vi "Finish.vi"   [LabVIEW 2018]
doc: "This VI is called just before exiting. It is expected to close I/O refnum, save collected data, etc."
uses:
  RefNums_DriverStation.vi
  RefNums_Actuators.vi
  RefNums_Sensors.vi
  <vilib>/Rock Robotics/WPI/Utilities/WPI_GetSetVariantRefNum.vi
types:
  T1 = typedef "WPI_AnalogChannelDevRef.ctl" = cluster{"DevStatus":errorcluster, "Analog Channel":T2}
  T2 = typedef "FPGA_AIChannel.ctl" = enum8{"AI 0", "AI 1", "AI 2", "AI 3", "AI MXP 0", "AI MXP 1", "AI MXP 2", "AI MXP 3", "Invalid"}
  T3 = typedef "WPI_RobotDriveDevRef.ctl" = cluster{"DevStatus":errorcluster, "Motors[]":T4[], "Square Inputs":bool, "Max Output":dbl}
  T4 = typedef "WPI_MotorControlDeviceRef.ctl" = cluster{"DeviceStatus":errorcluster, "Type":T5, "PWM":cluster{"PWM Channel":T6, "DeadBand":T7}, "CAN":cluster{"Device Number":u8, "SetOutput VI Ref":variant, "GetOutput VI Ref":variant, "Enable VI Ref":variant, "Disable VI Ref":variant, "Data":variant}, "Invert":bool, "DIO PWM":cluster{"PWM \"Enable\" Channel":T6, "DIOChannel":T8, "PWM Rate":dbl}}
  T5 = typedef "WPI_MotorControlType.ctl" = enum16{"PWM", "CAN", "DIO PWM"}
  T6 = typedef "FPGA_DIOPWMChannel.ctl" = enum8{"PWM 0", "PWM 1", "PWM 2", "PWM 3", "PWM 4", "PWM 5", "PWM 6", "PWM 7", "PWM 8", "PWM 9", "PWM MXP 0", "PWM MXP 1", "PWM MXP 2", "PWM MXP 3", "PWM MXP 4", "PWM MXP 5", "PWM MXP 6", "PWM MXP 7", "PWM MXP 8", "PWM MXP 9", "Invalid"}
  T7 = typedef "WPI_PWMDeadband.ctl" = cluster{"Name":string, "maxPositivePwm":i32, "minPositivePwm":i32, "centerPwm":i32, "maxNegativePwm":i32, "minNegativePwm":i32, "angularRange":u16}
  T8 = typedef "FPGA_DIOChannel.ctl" = enum8{"DIO 0", "DIO 1", "DIO 2", "DIO 3", "DIO 4", "DIO 5", "DIO 6", "DIO 7", "DIO 8", "DIO 9", "DIO MXP 0", "DIO MXP 1", "DIO MXP 2", "DIO MXP 3", "DIO MXP 4", "DIO MXP 5", "DIO MXP 6", "DIO MXP 7", "DIO MXP 8", "DIO MXP 9", "DIO MXP 10", "DIO MXP 11", "DIO MXP 12", "DIO MXP 13", "DIO MXP 14", "DIO MXP 15", "SPI Port CS1", "SPI Port CS2", "SPI Port CS3", "SPI Port MISO", "SPI Port MOSI", "Invalid"}
  T9 = typedef "WPI_ServoDeviceRef.ctl" = cluster{"DeviceStatus":errorcluster, "PWM Channel":T6, "DeadBand":T7}
  T10 = typedef "WPI_SolenoidDevRef.ctl" = cluster{"DevStatus":errorcluster, "Pneumatics Control Module":u8, "Forward Solenoid Channel":T11, "Reverse Solenoid Channel":T11}
  T11 = typedef "WPI_SolenoidChannel.ctl" = enum8{"Solenoid 0", "Solenoid 1", "Solenoid 2", "Solenoid 3", "Solenoid 4", "Solenoid 5", "Solenoid 6", "Solenoid 7", "Invalid"}
  T12 = typedef "WPI_JoystickDevRef.ctl" = cluster{"Device":T13}
  T13 = typedef "WPI_JoystickDeviceEnum.ctl" = enum16{"USB 0", "USB 1", "USB 2", "USB 3", "USB 4", "USB 5"}
  T14 = typedef "WPI_CompressorDevRef.ctl" = cluster{"DevStatus":errorcluster, "Pneumatics Control Module":u8}
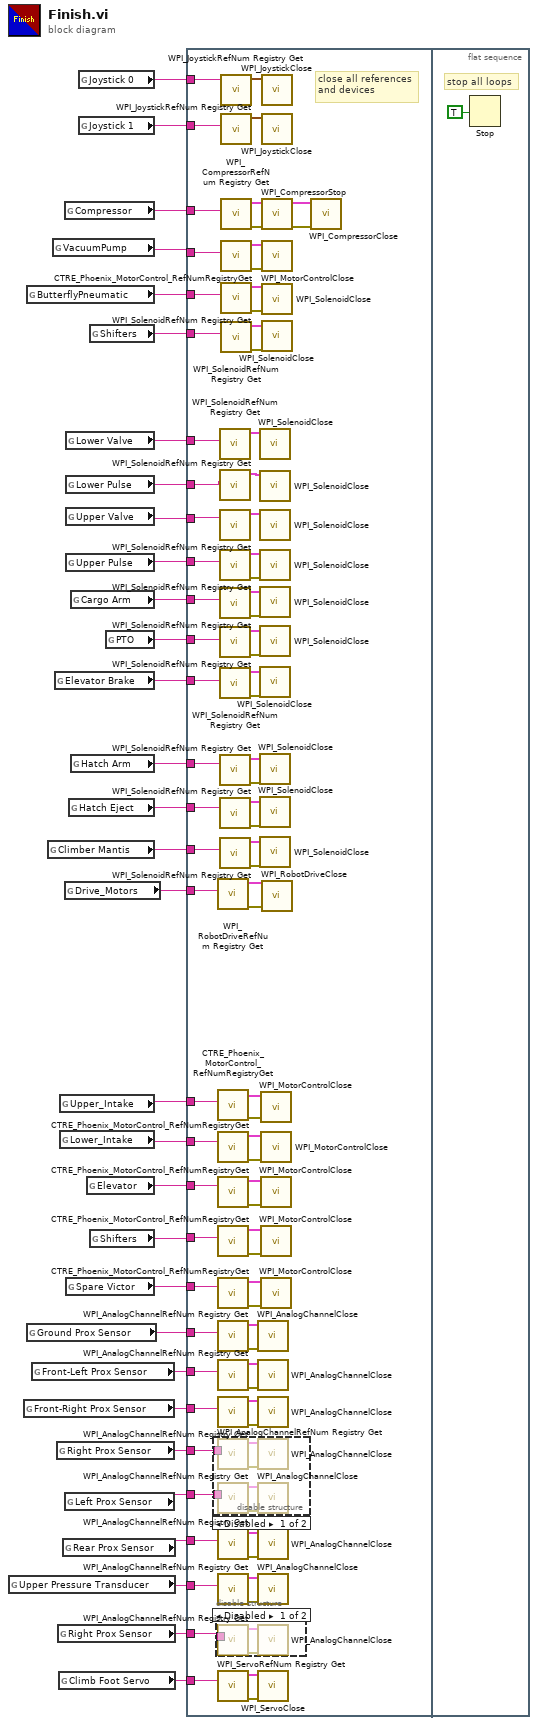
[diagram p0: block diagram]
diagram:
  n1 = global read "RefNums_Sensors.vi" "Upper Pressure Transducer"() -> (w18:string)
  n2 = global read "RefNums_Sensors.vi" "Front-Right Prox Sensor"() -> (w5:string)
  n3 = global read "RefNums_Actuators.vi" "ButterflyPneumatic"() -> (w28:string)
  n4 = global read "RefNums_Sensors.vi" "Ground Prox Sensor"() -> (w4:string)
  n5 = global read "RefNums_Sensors.vi" "Front-Left Prox Sensor"() -> (w6:string)
  n6 = global read "RefNums_Actuators.vi" "Climber Mantis"() -> (w10:string)
  n7 = global read "RefNums_Actuators.vi" "VacuumPump"() -> (w26:string)
  n8 = global read "RefNums_Actuators.vi" "Elevator Brake"() -> (w13:string)
  n9 = global read "RefNums_Sensors.vi" "Right Prox Sensor"() -> (w20:string)
  n10 = global read "RefNums_Sensors.vi" "Right Prox Sensor"() -> (w3:string)
  n11 = global read "RefNums_Actuators.vi" "Climb Foot Servo"() -> (w1:string)
  n12 = global read "RefNums_Actuators.vi" "Upper_Intake"() -> (w23:string)
  n13 = global read "RefNums_Actuators.vi" "Lower_Intake"() -> (w22:string)
  n14 = global read "RefNums_Sensors.vi" "Rear Prox Sensor"() -> (w17:string)
  n15 = global read "RefNums_Actuators.vi" "Compressor"() -> (w29:string)
  n16 = global read "RefNums_Actuators.vi" "Drive_Motors"() -> (w2:string)
  n17 = global read "RefNums_Sensors.vi" "Left Prox Sensor"() -> (w19:string)
  n18 = global read "RefNums_Actuators.vi" "Lower Valve"() -> (w8:string)
  n19 = global read "RefNums_Actuators.vi" "Lower Pulse"() -> (w7:string)
  n20 = global read "RefNums_Actuators.vi" "Upper Valve"() -> (w9:string)
  n21 = global read "RefNums_Actuators.vi" "Upper Pulse"() -> (w25:string)
  n22 = global read "RefNums_Actuators.vi" "Spare Victor"() -> (w15:string)
  n23 = global read "RefNums_Actuators.vi" "Hatch Eject"() -> (w11:string)
  n24 = global read "RefNums_Actuators.vi" "Cargo Arm"() -> (w24:string)
  n25 = global read "RefNums_Actuators.vi" "Hatch Arm"() -> (w12:string)
  n26 = global read "RefNums_DriverStation.vi" "Joystick 0"() -> (w30:string)
  n27 = global read "RefNums_DriverStation.vi" "Joystick 1"() -> (w31:string)
  n28 = global read "RefNums_Actuators.vi" "Elevator"() -> (w21:string)
  n29 = global read "RefNums_Actuators.vi" "Shifters"() -> (w27:string)
  n30 = global read "RefNums_Actuators.vi" "Shifters"() -> (w16:string)
  n31 = global read "RefNums_Actuators.vi" "PTO"() -> (w14:string)
  n32 = flat-sequence {
    tunnel: w31 -> [w114]
    tunnel: w30 -> [w115]
    tunnel: w29 -> [w111]
    tunnel: w28 -> [w110]
    tunnel: w27 -> [w105]
    tunnel: w26 -> [w104]
    tunnel: w25 -> [w102]
    tunnel: w24 -> [w99]
    tunnel: w23 -> [w97]
    tunnel: w22 -> [w95]
    tunnel: w21 -> [w93]
    tunnel: w20 -> [w92]
    tunnel: w19 -> [w77]
    tunnel: w17 -> [w76]
    tunnel: w18 -> [w75]
    tunnel: w16 -> [w72]
    tunnel: w15 -> [w70]
    tunnel: w14 -> [w64]
    tunnel: w13 -> [w63]
    tunnel: w12 -> [w56]
    tunnel: w11 -> [w55]
    tunnel: w10 -> [w54]
    tunnel: w9 -> [w50]
    tunnel: w8 -> [w49]
    tunnel: w7 -> [w48]
    tunnel: w6 -> [w43]
    tunnel: w5 -> [w42]
    tunnel: w4 -> [w39]
    tunnel: w3 -> [w38]
    tunnel: w2 -> [w35]
    tunnel: w1 -> [w34]
    frame #0 {
      # "close all references\nand devices"
      n33 = disable-structure shown="Disabled" {
        disable-tunnel: w92 -> [w123 _]
        disable-tunnel: w77 -> [w119 _]
        frame Disabled {
          n34 = call <vilib>:"WPI_AnalogChannelRefNum Registry Get.vi"("refnum name"=w123) -> ("error out"=w122:errorcluster, "AIDeviceRef"=w124:T1)  [unwired: 9 in]
          n35 = call <vilib>:"WPI_AnalogChannelRefNum Registry Get.vi"("refnum name"=w119) -> ("error out"=w120:errorcluster, "AIDeviceRef"=w121:T1)  [unwired: 9 in]
          n36 = call <vilib>:"WPI_AnalogChannelClose.vi"("error in (no error)"=w122, "AIDeviceRef"=w124) -> ()  [unwired: 9 in, 1 out]
          n37 = call <vilib>:"WPI_AnalogChannelClose.vi"("error in (no error)"=w120, "AIDeviceRef"=w121) -> ()  [unwired: 9 in, 1 out]
        }
        frame Enabled {
        }
      }
      n38 = disable-structure shown="Disabled" {
        disable-tunnel: w38 -> [w116 _]
        frame Disabled {
          n39 = call <vilib>:"WPI_AnalogChannelRefNum Registry Get.vi"("refnum name"=w116) -> ("error out"=w118:errorcluster, "AIDeviceRef"=w117:T1)  [unwired: 9 in]
          n40 = call <vilib>:"WPI_AnalogChannelClose.vi"("error in (no error)"=w118, "AIDeviceRef"=w117) -> ()  [unwired: 9 in, 1 out]
        }
        frame Enabled {
        }
      }
      n41 = call <vilib>:"WPI_RobotDriveRefNum Registry Get.vi"("refnum name"=w35) -> ("error out"=w37:errorcluster, "RobotDriveDevRef"=w36:T3)  [unwired: 9 in]
      n42 = call <vilib>:"CTRE_Phoenix_MotorControl_RefNumRegistryGet.vi"("refnum name"=w97) -> ("error out"=w89:errorcluster, "PhoenixMotorControlDevRef"=w98:T4)  [unwired: 9 in]
      n43 = call <vilib>:"CTRE_Phoenix_MotorControl_RefNumRegistryGet.vi"("refnum name"=w95) -> ("error out"=w90:errorcluster, "PhoenixMotorControlDevRef"=w96:T4)  [unwired: 9 in]
      n44 = call <vilib>:"CTRE_Phoenix_MotorControl_RefNumRegistryGet.vi"("refnum name"=w93) -> ("error out"=w91:errorcluster, "PhoenixMotorControlDevRef"=w94:T4)  [unwired: 9 in]
      n45 = call <vilib>:"CTRE_Phoenix_MotorControl_RefNumRegistryGet.vi"("refnum name"=w72) -> ("error out"=w74:errorcluster, "PhoenixMotorControlDevRef"=w73:T4)  [unwired: 9 in]
      n46 = call <vilib>:"CTRE_Phoenix_MotorControl_RefNumRegistryGet.vi"("refnum name"=w70) -> ("error out"=w71:errorcluster, "PhoenixMotorControlDevRef"=w69:T4)  [unwired: 9 in]
      n47 = call <vilib>:"WPI_AnalogChannelRefNum Registry Get.vi"("refnum name"=w39) -> ("error out"=w40:errorcluster, "AIDeviceRef"=w41:T1)  [unwired: 9 in]
      n48 = call <vilib>:"WPI_AnalogChannelRefNum Registry Get.vi"("refnum name"=w43) -> ("error out"=w44:errorcluster, "AIDeviceRef"=w45:T1)  [unwired: 9 in]
      n49 = call <vilib>:"WPI_AnalogChannelRefNum Registry Get.vi"("refnum name"=w42) -> ("error out"=w46:errorcluster, "AIDeviceRef"=w47:T1)  [unwired: 9 in]
      n50 = call <vilib>:"WPI_AnalogChannelRefNum Registry Get.vi"("refnum name"=w76) -> ("error out"=w80:errorcluster, "AIDeviceRef"=w81:T1)  [unwired: 9 in]
      n51 = call <vilib>:"WPI_AnalogChannelRefNum Registry Get.vi"("refnum name"=w75) -> ("error out"=w78:errorcluster, "AIDeviceRef"=w79:T1)  [unwired: 9 in]
      n52 = call <vilib>:"WPI_ServoRefNum Registry Get.vi"("refnum name"=w34) -> ("error out"=w33:errorcluster, "ServoDeviceRef"=w32:T9)  [unwired: 9 in]
      n53 = call <vilib>:"WPI_SolenoidRefNum Registry Get.vi"("refnum name"=w49) -> ("SolenoidDevRef"=w53:T10)  [unwired: 9 in, 1 out]
      n54 = call <vilib>:"WPI_SolenoidRefNum Registry Get.vi"("refnum name"=w48) -> ("SolenoidDevRef"=w52:T10)  [unwired: 9 in, 1 out]
      n55 = call <vilib>:"WPI_SolenoidRefNum Registry Get.vi"("refnum name"=w50) -> ("SolenoidDevRef"=w51:T10)  [unwired: 9 in, 1 out]
      n56 = call <vilib>:"WPI_SolenoidRefNum Registry Get.vi"("refnum name"=w102) -> ("error out"=w87:errorcluster, "SolenoidDevRef"=w101:T10)  [unwired: 9 in]
      n57 = call <vilib>:"WPI_SolenoidRefNum Registry Get.vi"("refnum name"=w99) -> ("error out"=w88:errorcluster, "SolenoidDevRef"=w100:T10)  [unwired: 9 in]
      n58 = call <vilib>:"WPI_SolenoidRefNum Registry Get.vi"("refnum name"=w64) -> ("error out"=w67:errorcluster, "SolenoidDevRef"=w68:T10)  [unwired: 9 in]
      n59 = call <vilib>:"WPI_SolenoidRefNum Registry Get.vi"("refnum name"=w63) -> ("error out"=w65:errorcluster, "SolenoidDevRef"=w66:T10)  [unwired: 9 in]
      n60 = call <vilib>:"WPI_SolenoidRefNum Registry Get.vi"("refnum name"=w56) -> ("error out"=w61:errorcluster, "SolenoidDevRef"=w62:T10)  [unwired: 9 in]
      n61 = call <vilib>:"WPI_SolenoidRefNum Registry Get.vi"("refnum name"=w55) -> ("error out"=w59:errorcluster, "SolenoidDevRef"=w60:T10)  [unwired: 9 in]
      n62 = call <vilib>:"WPI_SolenoidRefNum Registry Get.vi"("refnum name"=w54) -> ("error out"=w57:errorcluster, "SolenoidDevRef"=w58:T10)  [unwired: 9 in]
      n63 = call <vilib>:"WPI_JoystickRefNum Registry Get.vi"("refnum name"=w115) -> ("JoystickDevRef"=w112:T12)  [unwired: 9 in, 1 out]
      n64 = call <vilib>:"WPI_JoystickRefNum Registry Get.vi"("refnum name"=w114) -> ("JoystickDevRef"=w113:T12)  [unwired: 9 in, 1 out]
      n65 = call <vilib>:"WPI_CompressorRefNum Registry Get.vi"("refnum name"=w111) -> ("error out"=w83:errorcluster, "CompressorDevRef"=w108:T14)  [unwired: 9 in]
      n66 = call <vilib>:"CTRE_Phoenix_MotorControl_RefNumRegistryGet.vi"("refnum name"=w104) -> ("error out"=w84:errorcluster, "PhoenixMotorControlDevRef"=w103:T4)  [unwired: 9 in]
      n67 = call <vilib>:"WPI_SolenoidRefNum Registry Get.vi"("refnum name"=w110) -> ("error out"=w85:errorcluster, "SolenoidDevRef"=w109:T10)  [unwired: 9 in]
      n68 = call <vilib>:"WPI_SolenoidRefNum Registry Get.vi"("refnum name"=w105) -> ("error out"=w86:errorcluster, "SolenoidDevRef"=w106:T10)  [unwired: 9 in]
      n69 = call <vilib>:"WPI_AnalogChannelClose.vi"("error in (no error)"=w40, "AIDeviceRef"=w41) -> ()  [unwired: 9 in, 1 out]
      n70 = call <vilib>:"WPI_AnalogChannelClose.vi"("error in (no error)"=w44, "AIDeviceRef"=w45) -> ()  [unwired: 9 in, 1 out]
      n71 = call <vilib>:"WPI_AnalogChannelClose.vi"("error in (no error)"=w46, "AIDeviceRef"=w47) -> ()  [unwired: 9 in, 1 out]
      n72 = call <vilib>:"WPI_AnalogChannelClose.vi"("error in (no error)"=w80, "AIDeviceRef"=w81) -> ()  [unwired: 9 in, 1 out]
      n73 = call <vilib>:"WPI_AnalogChannelClose.vi"("error in (no error)"=w78, "AIDeviceRef"=w79) -> ()  [unwired: 9 in, 1 out]
      n74 = call <vilib>:"WPI_ServoClose.vi"("error in (no error)"=w33, "ServoDeviceRef"=w32) -> ()  [unwired: 9 in, 1 out]
      n75 = call <vilib>:"WPI_SolenoidClose.vi"("SolenoidDevRef"=w53) -> ()  [unwired: 10 in, 1 out]
      n76 = call <vilib>:"WPI_SolenoidClose.vi"("SolenoidDevRef"=w52) -> ()  [unwired: 10 in, 1 out]
      n77 = call <vilib>:"WPI_SolenoidClose.vi"("SolenoidDevRef"=w51) -> ()  [unwired: 10 in, 1 out]
      n78 = call <vilib>:"WPI_SolenoidClose.vi"("error in (no error)"=w87, "SolenoidDevRef"=w101) -> ()  [unwired: 9 in, 1 out]
      n79 = call <vilib>:"WPI_SolenoidClose.vi"("error in (no error)"=w88, "SolenoidDevRef"=w100) -> ()  [unwired: 9 in, 1 out]
      n80 = call <vilib>:"WPI_SolenoidClose.vi"("error in (no error)"=w67, "SolenoidDevRef"=w68) -> ()  [unwired: 9 in, 1 out]
      n81 = call <vilib>:"WPI_SolenoidClose.vi"("error in (no error)"=w65, "SolenoidDevRef"=w66) -> ()  [unwired: 9 in, 1 out]
      n82 = call <vilib>:"WPI_SolenoidClose.vi"("error in (no error)"=w61, "SolenoidDevRef"=w62) -> ()  [unwired: 9 in, 1 out]
      n83 = call <vilib>:"WPI_SolenoidClose.vi"("error in (no error)"=w59, "SolenoidDevRef"=w60) -> ()  [unwired: 9 in, 1 out]
      n84 = call <vilib>:"WPI_SolenoidClose.vi"("error in (no error)"=w57, "SolenoidDevRef"=w58) -> ()  [unwired: 9 in, 1 out]
      n85 = call <vilib>:"WPI_MotorControlClose.vi"("error in"=w89, "MotorControlDevRef"=w98) -> ()  [unwired: 9 in, 1 out]
      n86 = call <vilib>:"WPI_MotorControlClose.vi"("error in"=w90, "MotorControlDevRef"=w96) -> ()  [unwired: 9 in, 1 out]
      n87 = call <vilib>:"WPI_MotorControlClose.vi"("error in"=w91, "MotorControlDevRef"=w94) -> ()  [unwired: 9 in, 1 out]
      n88 = call <vilib>:"WPI_MotorControlClose.vi"("error in"=w74, "MotorControlDevRef"=w73) -> ()  [unwired: 9 in, 1 out]
      n89 = call <vilib>:"WPI_MotorControlClose.vi"("error in"=w71, "MotorControlDevRef"=w69) -> ()  [unwired: 9 in, 1 out]
      n90 = call <vilib>:"WPI_JoystickClose.vi"("JoystickDevRef"=w112) -> ()  [unwired: 11 in]
      n91 = call <vilib>:"WPI_JoystickClose.vi"("JoystickDevRef"=w113) -> ()  [unwired: 11 in]
      n92 = call <vilib>:"WPI_CompressorStop.vi"("error in (no error)"=w83, "CompressorDevRef"=w108) -> ("error out"=w82:errorcluster, "CompressorDevRef"=w107:T14)  [unwired: 8 in]
      n93 = call <vilib>:"WPI_MotorControlClose.vi"("error in"=w84, "MotorControlDevRef"=w103) -> ()  [unwired: 9 in, 1 out]
      n94 = call <vilib>:"WPI_SolenoidClose.vi"("error in (no error)"=w85, "SolenoidDevRef"=w109) -> ()  [unwired: 9 in, 1 out]
      n95 = call <vilib>:"WPI_SolenoidClose.vi"("error in (no error)"=w86, "SolenoidDevRef"=w106) -> ()  [unwired: 9 in, 1 out]
      n96 = call <vilib>:"WPI_RobotDriveClose.vi"("error in (no error)"=w37, "RobotDriveDevRef"=w36) -> ()  [unwired: 9 in, 1 out]
      n97 = call <vilib>:"WPI_CompressorClose.vi"("error in (no error)"=w82, "CompressorDevRef"=w107) -> ()  [unwired: 9 in, 1 out]
    }
    frame #1 {
      # "stop all loops"
      n98 = Stop(stop? (T)=TRUE ("Quit")) -> ()
    }
  }
